vi "Updated Command Processor Status.vi"(8 "error in (no error)":errorcluster, 10 "Command Processor Status":T1 {"Commands Behind" scale=0.0..10.0; "Queued Commands" scale=0.0..100.0}, 11 "System Actor in":refnum<class "System Actor.lvclass">) -> (0 "error out":errorcluster, 3 "System Actor out":refnum<class "System Actor.lvclass">)   [LabVIEW 2014, in "Robot Actor Framework.lvlib" / "System Actor.lvlib" / "System Actor.lvclass"]
uses:
  System Actor.lvclass
  Command Processor Actor/Command Processor Actor Class/Command Processor State.ctl
  Command Processor Actor/Command Processor Actor Class/Command Processor States.ctl
  Command Actor/Command Actor Class/Command State.ctl
  Command Actor/Command Actor Class/Command States.ctl
  Command Processor Actor/Command Processor Actor Class/Command Processor Actor.lvclass
  Command Actor/Command Actor Class/Command Actor.lvclass
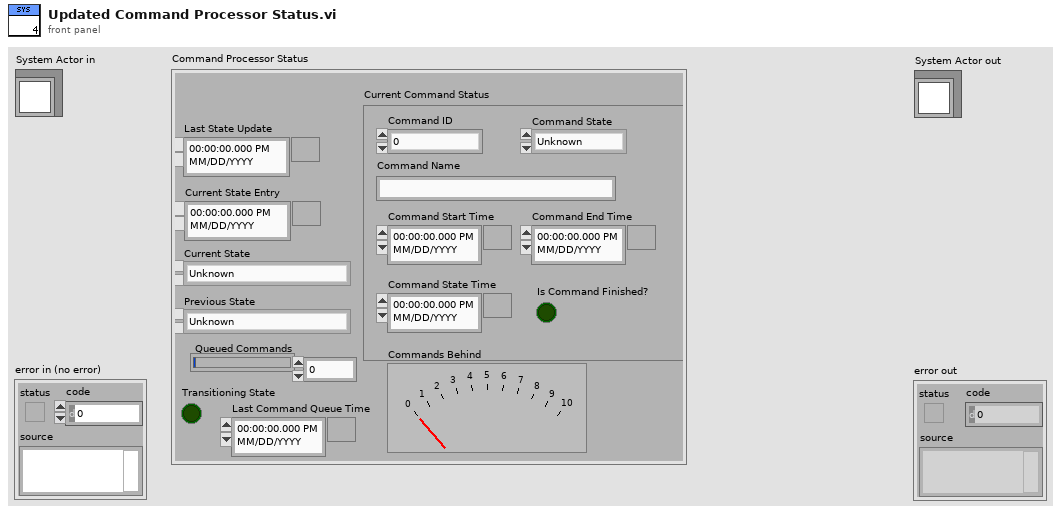
[diagram p1: front panel]
types:
  T1 = typedef "Robot Actor Framework.lvlib/Command Processor Actor.lvlib/Command Processor Actor.lvclass/Command Processor State.ctl" = cluster{"Current State":T2, "Last State Update":timestamp, "Queued Commands":u32, "Current Command Status":T3, "Previous State":T2, "Current State Entry":timestamp, "Transitioning State":bool, "Commands Behind":dbl, "Last Command Queue Time":timestamp}
  T2 = typedef "Robot Actor Framework.lvlib/Command Processor Actor.lvlib/Command Processor Actor.lvclass/Command Processor States.ctl" = enum16{"Unknown", "No Command", "Running Command", "Starting Command", "Stopping Command", "Finishing Command"}
  T3 = typedef "Robot Actor Framework.lvlib/Command Actor.lvlib/Command Actor.lvclass/Command State.ctl" = cluster{"Command Name":string, "Command Start Time":timestamp, "Command End Time":timestamp, "Is Command Finished?":bool, "Command ID":u32, "Command State":T4, "Command State Time":timestamp}
  T4 = typedef "Robot Actor Framework.lvlib/Command Actor.lvlib/Command Actor.lvclass/Command States.ctl" = enum16{"Unknown", "Started", "Stopped", "Finished"}
  T5 = typedef "Robot Actor Framework.lvlib/System Actor.lvlib/System Actor.lvclass/System State.ctl" = cluster{"Instance Name":string, "Current Command Status":T3, "System Start Time":timestamp, "Next Command ID":dbl, "Command Processor Status":T1}
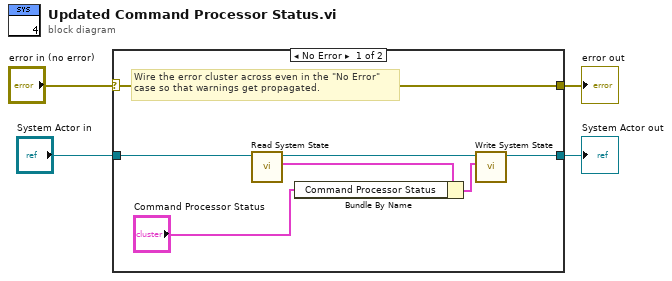
[diagram p0: block diagram]
diagram:
  n1 = case shown="No Error" "error in (no error)" {
    selector: "error in (no error)" -> [w11 w13]
    tunnel: [w11 w13] -> w3
    tunnel: [w8 w12] -> w1
    tunnel: "System Actor in" -> [w10 w12]
    frame No Error {
      # "Wire the error cluster across even in the \"No Error\"\ncase so that warnings get propagated."
      n2 = call-dynamic "Read System State.vi"("System Actor in"=w10) -> ("System Status"=w7:T5, "System Actor out"=w9:refnum<class "System Actor.lvclass">)  [unwired: 8 in, 1 out]
      n3 = Bundle By Name(cluster=w7, "Command Processor Status"="Command Processor Status") -> (w6:T5)
      n4 = call-dynamic "Write System State.vi"("System Status"=w6, "System Actor in"=w9) -> ("System Actor out"=w8:refnum<class "System Actor.lvclass">)  [unwired: 8 in, 1 out]
    }
    frame Error {
    }
  }
  "error out" <- w3
  "System Actor out" <- w1
